vi "Actor Core.vi"(8 "error in":errorcluster, 11 "HardwareSetup_modle001:HardwareSetup_modle001":refnum<class "HardwareSetup_model001.lvclass">) -> (0 "error out":errorcluster, 3 "HardwareSetup_modle001:HardwareSetup_modle001":refnum<class "Actor.lvclass">)   [LabVIEW 2019, in "HardwareSetup_model001.lvlib" / "HardwareSetup_model001.lvclass"]
doc: "(<B>Filename</B>: Actor Framework.lvlib:Actor.lvclass:Actor Core.vi)\n\nReceives messages to the actor, reacts to them, and initiates any error handling that may shut the actor down.\n\nDescendant classes may override this VI to append parallel tasks for the actor to complete while it handles messages. Overrides use the Call Parent Method node."
uses:
  HardwareSetup_model001.lvclass
  PLC.ctl
  LIN.ctl
  CAN.ctl
  Programming.ctl
  DMM.ctl
  Scanner.ctl
  ElectronicLoad.ctl
  Oscilloscope.ctl
  Digital IO.ctl
  C:/Program Files (x86)/National Instruments/LabVIEW 2019/vi.lib/ActorFramework/Actor/Actor.lvclass
  <vilib>/ActorFramework/Actor/Actor.lvclass
  PowerSupply.ctl
  HardwareSetup_model001.lvclass/HardwareSetup_model001.ctl
  <vilib>/ActorFramework/Actor/Actor.lvclass/Actor.ctl
  <vilib>/ActorFramework/Message Enqueuer/Message Enqueuer.lvclass/Message Enqueuer.ctl
  2d133038-814c-4d09-b03d-156015606240.vi
  <vilib>/ActorFramework/Message Enqueuer/Init from Existing Queue.vi
  <vilib>/ActorFramework/Message Enqueuer/Enqueue.vi
  SystemSetup/SystemSetup Messages/RefreshSystemConfigurationUI Msg/RefreshSystemConfigurationUI Msg.lvclass
  C:/Program Files (x86)/National Instruments/LabVIEW 2019/vi.lib/ActorFramework/Message/Message.lvclass
  SystemSetup/SystemSetup Messages/SaveSystemConfigurationUI Msg/SaveSystemConfigurationUI Msg.lvclass
  <vilib>/ActorFramework/Message Priority Queue/Priority Enqueue.vi
  <vilib>/ActorFramework/Message Enqueuer/Message Enqueuer.lvclass
  SystemSetup/SystemSetup/SystemSetup.lvclass
  b9caf896-7e68-41be-8993-ec1cdb98c7cc.vi
  HardwareSetup_model001.lvlib
panel:
  in  "Tab Control":T1(tab)
  in  "PowerSupply":T2
  in  "Digital IO":T3
  in  "Oscilloscope":T4
  in  "ElectronicLoad":T5
  in  "Scanner":T6
  in  "DMM":T7
  in  "PLC":T8
  in  "CAN":T9
  in  "LIN":T10
  in  "Programming":T11
  in  "OK":bool
  in  "Cancel":bool
  # "PowerSupply_4"
  # "PowerSupply_3"
  # "PowerSupply_2"
  # "PowerSupply_1"
  # "Digital IO_4"
  # "Digital IO_3"
  # "Digital IO_2"
  # "Digital IO_1"
  # "Oscilloscope_4"
  # "Oscilloscope_3"
  # "Oscilloscope_2"
  # "Oscilloscope_1"
  # "ElectronicLoad_4"
  # "ElectronicLoad_3"
  # "ElectronicLoad_2"
  # "ElectronicLoad_1"
  # "Scanner_4"
  # "Scanner_3"
  # "Scanner_2"
  # "Scanner_1"
  # "DMM_4"
  # "DMM_3"
  # "DMM_2"
  # "DMM_1"
  # "PLC_1"
  # "CAN_4"
  # "CAN_3"
  # "CAN_2"
  # "CAN_1"
  # "LIN_4"
  # "LIN_3"
  # "LIN_2"
  # "LIN_1"
  # "Programming_1"
  # "Programming_1"
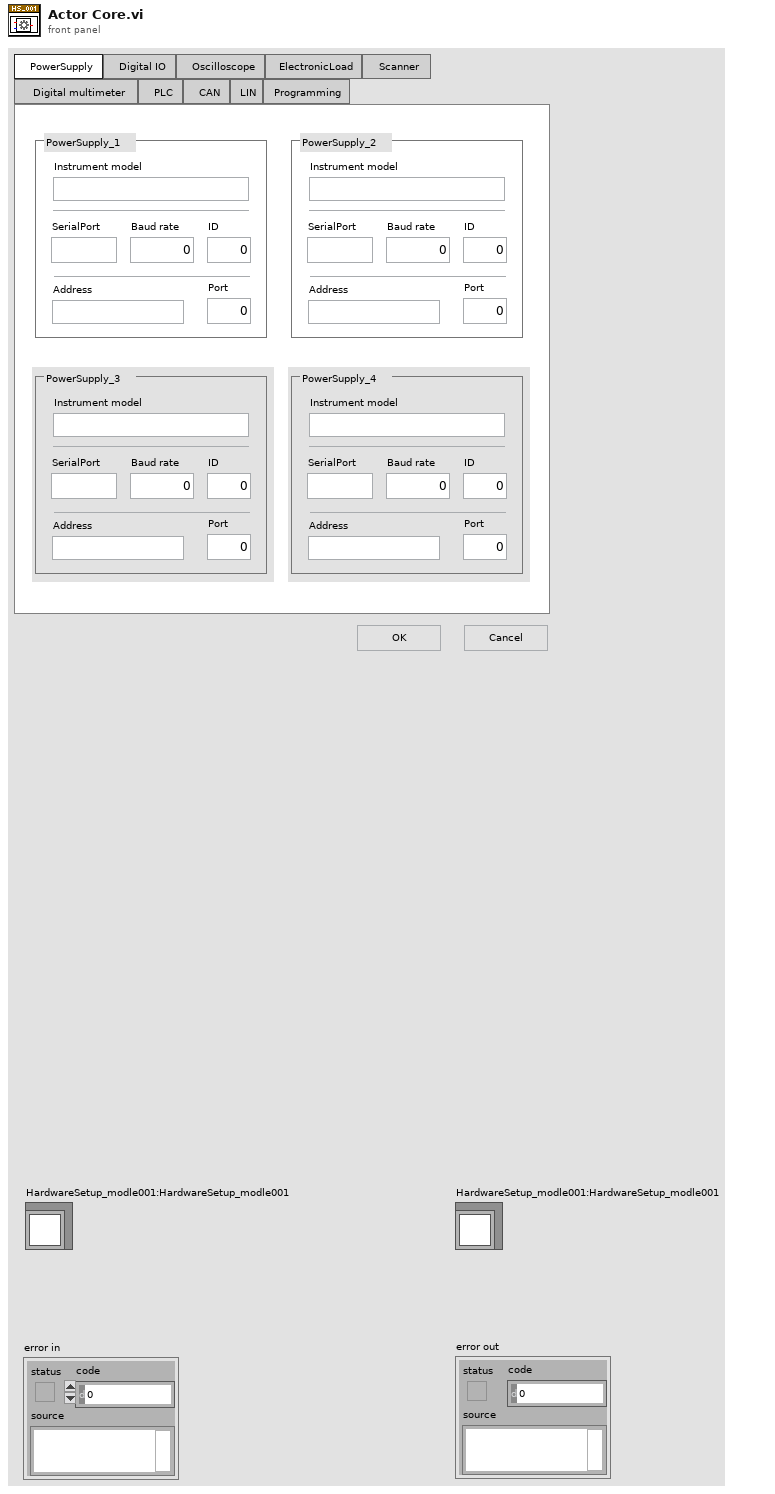
[diagram p1: front panel]
types:
  T1 = enum32{"  PowerSupply  ", "  Digital IO  ", "  Oscilloscope  ", "  ElectronicLoad ", "  Scanner   ", "  Digital multimeter    ", "  PLC  ", "  CAN  ", " LIN", " Programming "}
  T2 = typedef "HardwareSetup_model001.lvlib/PowerSupply.ctl" = cluster{"PowerSupply 1":cluster{"SerialPort":string, "Baud rate":i32, "Address":string, "ID":i32, "Port":i32, "Instrument model":string}, "PowerSupply 2":cluster{"SerialPort":string, "Baud rate":i32, "Address":string, "ID":i32, "Port":i32, "Instrument model":string}, "PowerSupply 3":cluster{"SerialPort":string, "Baud rate":i32, "Address":string, "ID":i32, "Port":i32, "Instrument model":string}, "PowerSupply 4":cluster{"SerialPort":string, "Baud rate":i32, "Address":string, "ID":i32, "Port":i32, "Instrument model":string}}
  T3 = typedef "HardwareSetup_model001.lvlib/Digital IO.ctl" = cluster{"Digital IO 1":cluster{"SerialPort":string, "Baud rate":i32, "Address":string, "ID":i32, "Port":i32, "Instrument model":string}, "Digital IO 2":cluster{"SerialPort":string, "Baud rate":i32, "Address":string, "ID":i32, "Port":i32, "Instrument model":string}, "Digital IO 3":cluster{"SerialPort":string, "Baud rate":i32, "Address":string, "ID":i32, "Port":i32, "Instrument model":string}, "Digital IO 4":cluster{"SerialPort":string, "Baud rate":i32, "Address":string, "ID":i32, "Port":i32, "Instrument model":string}}
  T4 = typedef "HardwareSetup_model001.lvlib/Oscilloscope.ctl" = cluster{"Oscilloscope 1":cluster{"SerialPort":string, "Baud rate":i32, "Address":string, "ID":i32, "Port":i32, "Instrument model":string}, "Oscilloscope 2":cluster{"SerialPort":string, "Baud rate":i32, "Address":string, "ID":i32, "Port":i32, "Instrument model":string}, "Oscilloscope 3":cluster{"SerialPort":string, "Baud rate":i32, "Address":string, "ID":i32, "Port":i32, "Instrument model":string}, "Oscilloscope 4":cluster{"SerialPort":string, "Baud rate":i32, "Address":string, "ID":i32, "Port":i32, "Instrument model":string}}
  T5 = typedef "HardwareSetup_model001.lvlib/ElectronicLoad.ctl" = cluster{"ElectronicLoad 1":cluster{"SerialPort":string, "Baud rate":i32, "Address":string, "ID":i32, "Port":i32, "Instrument model":string}, "ElectronicLoad 2":cluster{"SerialPort":string, "Baud rate":i32, "Address":string, "ID":i32, "Port":i32, "Instrument model":string}, "ElectronicLoad 3":cluster{"SerialPort":string, "Baud rate":i32, "Address":string, "ID":i32, "Port":i32, "Instrument model":string}, "ElectronicLoad 4":cluster{"SerialPort":string, "Baud rate":i32, "Address":string, "ID":i32, "Port":i32, "Instrument model":string}}
  T6 = typedef "HardwareSetup_model001.lvlib/Scanner.ctl" = cluster{"Scanner 1":cluster{"SerialPort":string, "Baud rate":i32, "Address":string, "ID":i32, "Port":i32, "Instrument model":string}, "Scanner 2":cluster{"SerialPort":string, "Baud rate":i32, "Address":string, "ID":i32, "Port":i32, "Instrument model":string}, "Scanner 3":cluster{"SerialPort":string, "Baud rate":i32, "Address":string, "ID":i32, "Port":i32, "Instrument model":string}, "Scanner 4":cluster{"SerialPort":string, "Baud rate":i32, "Address":string, "ID":i32, "Port":i32, "Instrument model":string}}
  T7 = typedef "HardwareSetup_model001.lvlib/DMM.ctl" = cluster{"DMM 1":cluster{"SerialPort":string, "Baud rate":i32, "Address":string, "ID":i32, "Port":i32, "Instrument model":string}, "DMM 2":cluster{"SerialPort":string, "Baud rate":i32, "Address":string, "ID":i32, "Port":i32, "Instrument model":string}, "DMM 3":cluster{"SerialPort":string, "Baud rate":i32, "Address":string, "ID":i32, "Port":i32, "Instrument model":string}, "DMM 4":cluster{"SerialPort":string, "Baud rate":i32, "Address":string, "ID":i32, "Port":i32, "Instrument model":string}}
  T8 = typedef "HardwareSetup_model001.lvlib/PLC.ctl" = cluster{"PLC 1":cluster{"SerialPort":string, "Baud rate":i32, "Address":string, "ID":i32, "Port":i32, "Instrument model":string}}
  T9 = typedef "HardwareSetup_model001.lvlib/CAN.ctl" = cluster{"CAN 1":cluster{"Instrument model":string, "Port":string, "Baud rate":i32, "ID":i32, "Terminal":bool}, "CAN 2":cluster{"Instrument model":string, "Port":string, "Baud rate":i32, "ID":i32, "Terminal":bool}, "CAN 3":cluster{"Instrument model":string, "Port":string, "Baud rate":i32, "ID":i32, "Terminal":bool}, "CAN 4":cluster{"Instrument model":string, "Port":string, "Baud rate":i32, "ID":i32, "Terminal":bool}}
  T10 = typedef "HardwareSetup_model001.lvlib/LIN.ctl" = cluster{"LIN 1":cluster{"Instrument model":string, "Port":string, "Baud rate":i32, "ID":i32, "Terminal":bool}, "LIN 2":cluster{"Instrument model":string, "Port":string, "Baud rate":i32, "ID":i32, "Terminal":bool}, "LIN 3":cluster{"Instrument model":string, "Port":string, "Baud rate":i32, "ID":i32, "Terminal":bool}, "LIN 4":cluster{"Instrument model":string, "Port":string, "Baud rate":i32, "ID":i32, "Terminal":bool}}
  T11 = typedef "HardwareSetup_model001.lvlib/Programming.ctl" = cluster{"Programming 1":cluster{"Test Image":string, "Address":string, "Port":i32, "Instrument model":string, "Final Image":string}, "Programming 2":cluster{"Test Image":string, "Address":string, "Port":i32, "Instrument model":string, "Final Image":string}}
  T12 = enum32{"Invalid", "Standard", "Closed", "Hidden", "Minimized", "Maximized"}
  T13 = enum32{"invalid app kind", "Development System", "Run Time System", "Student Edition", "Embedded LabVIEW", "Evaluation", "Custom"}
  T14 = cluster{"Core":cluster{"Current VI Reference":refnum<vi>, "Close Panel on Exit?":bool}, "Your Boolean data":bool, "Your string data":string}
  T15 = cluster{"Current VI Reference":refnum<vi>, "Close Panel on Exit?":bool}
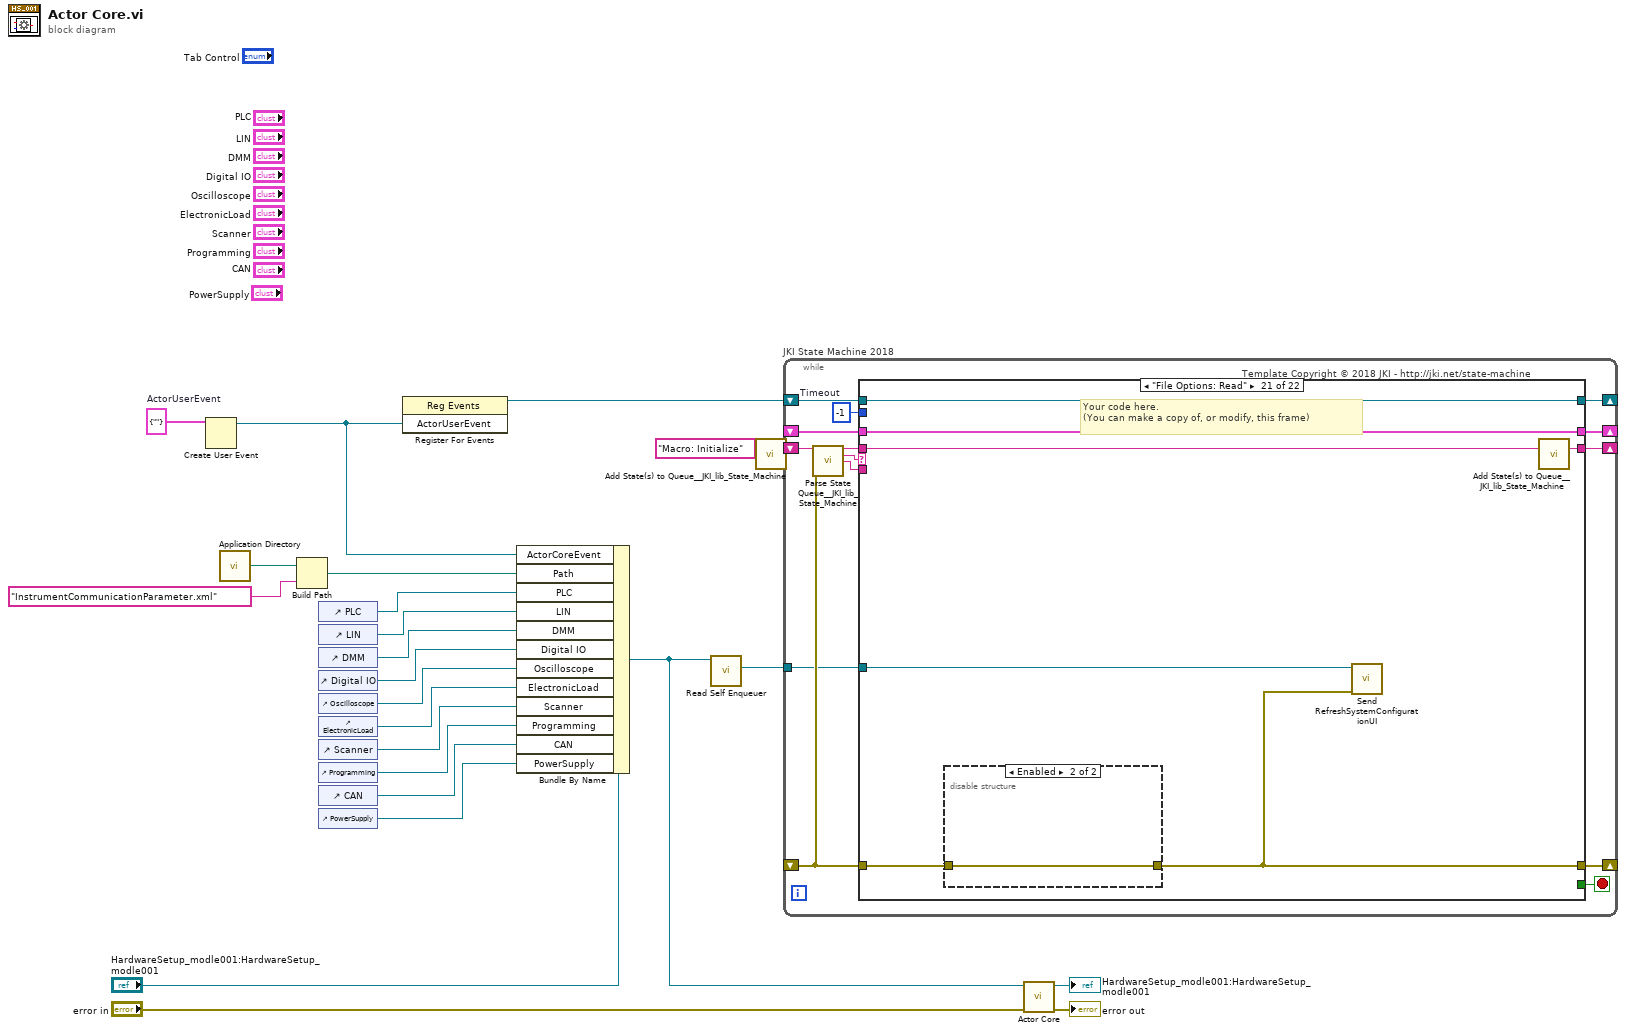
[diagram p0: block diagram]
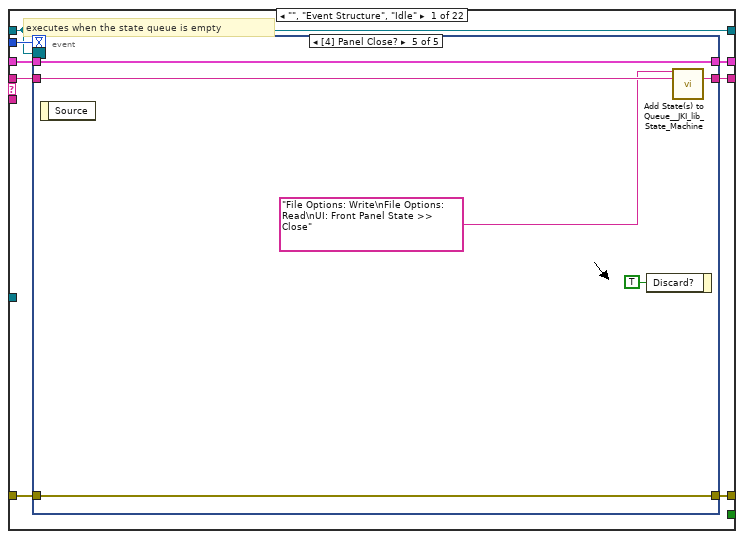
[diagram p2: hidden frame]
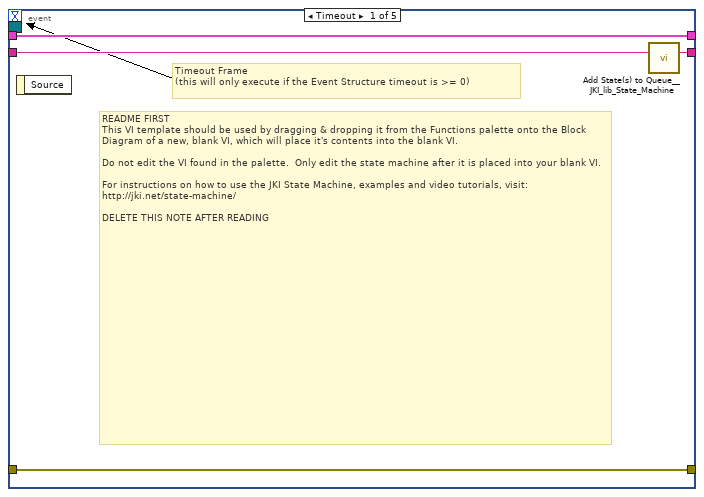
[diagram p3: hidden frame]
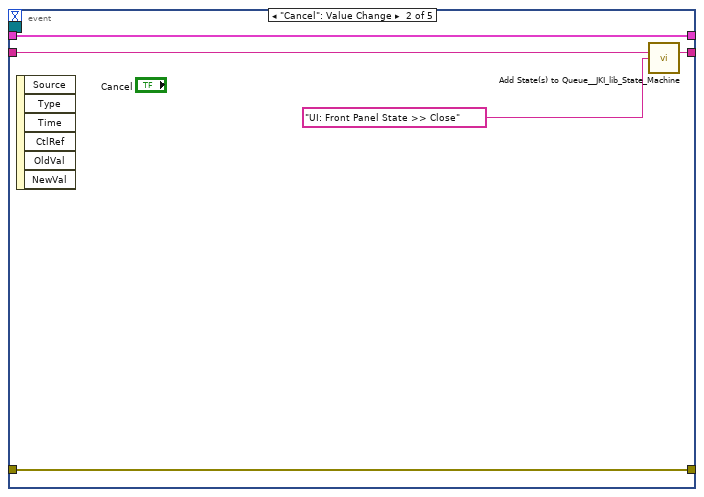
[diagram p4: hidden frame]
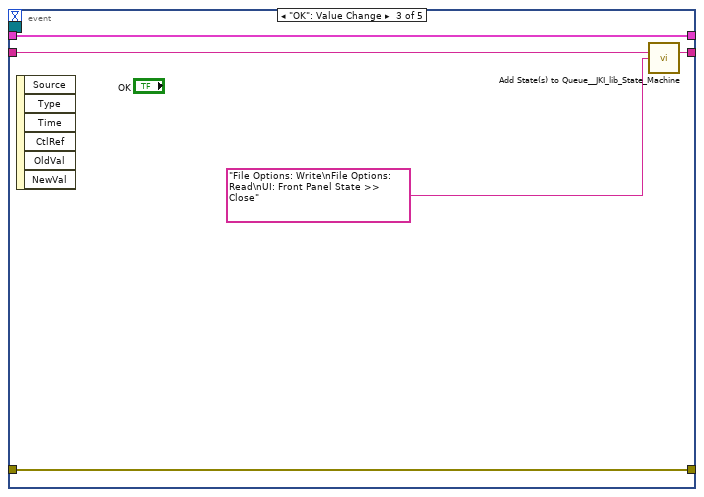
[diagram p5: hidden frame]
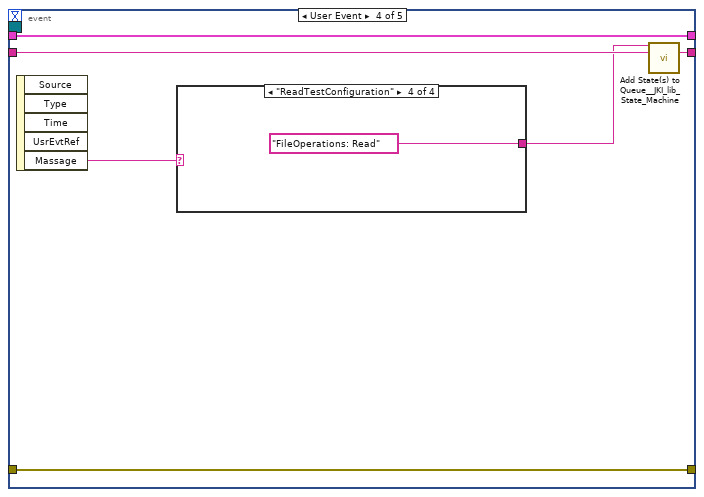
[diagram p6: hidden frame]
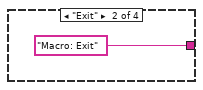
[diagram p8: hidden frame]
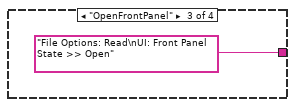
[diagram p9: hidden frame]
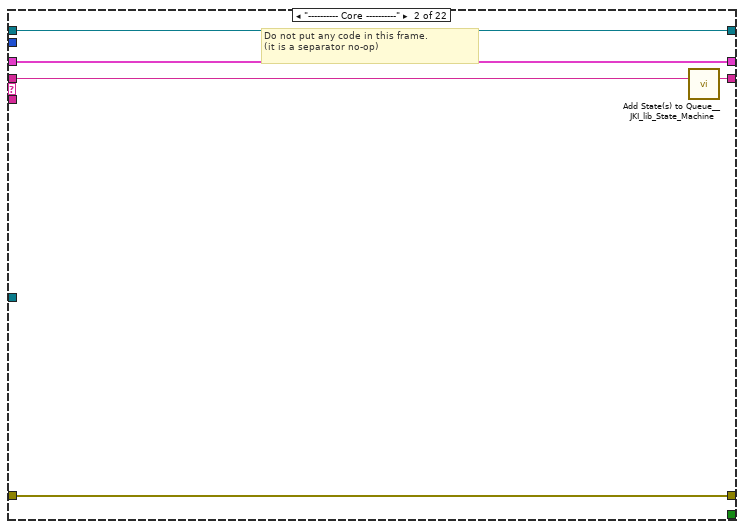
[diagram p10: hidden frame]
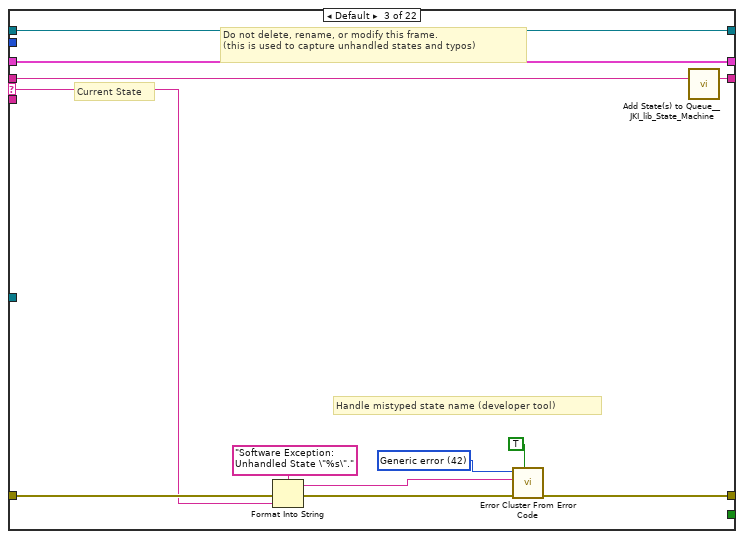
[diagram p11: hidden frame]
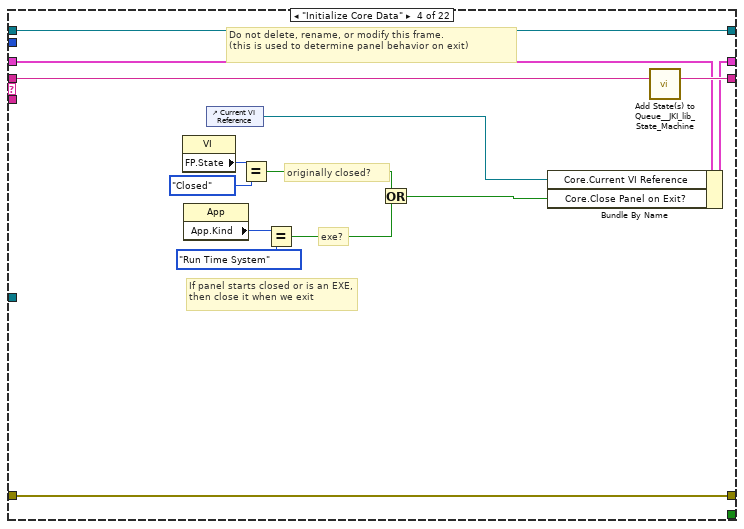
[diagram p12: hidden frame]
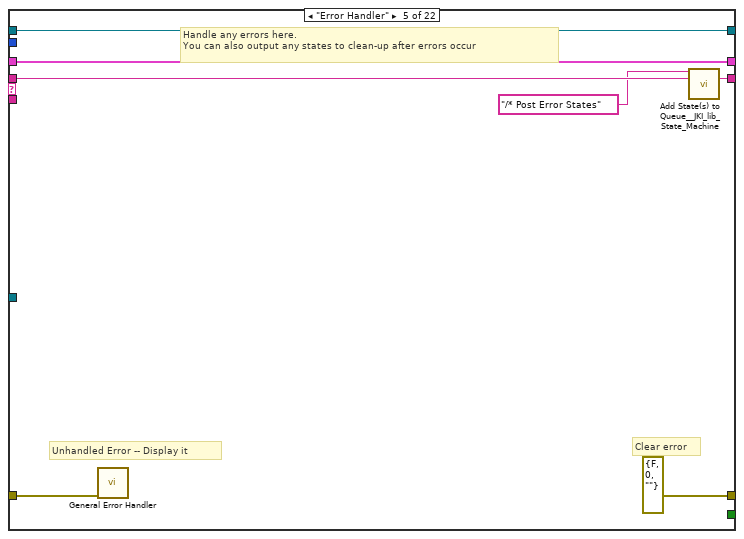
[diagram p13: hidden frame]
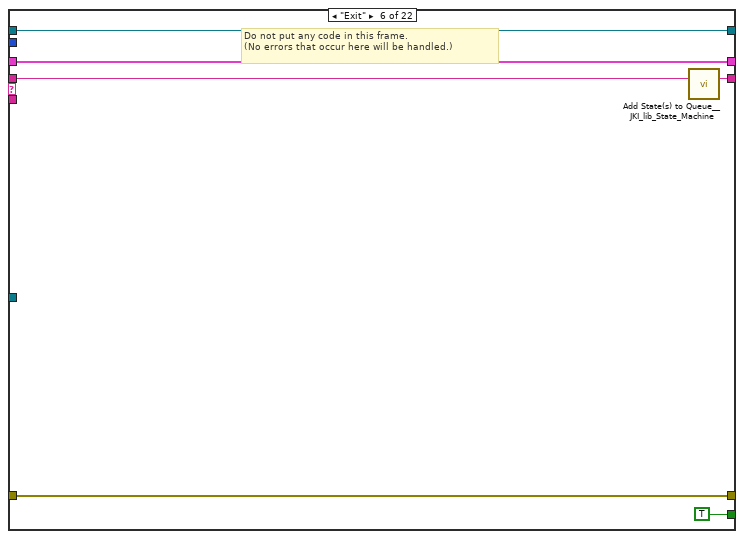
[diagram p14: hidden frame]
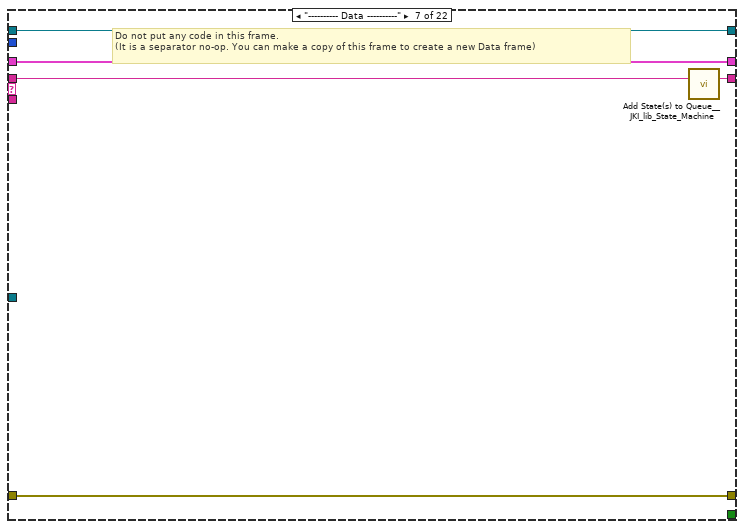
[diagram p15: hidden frame]
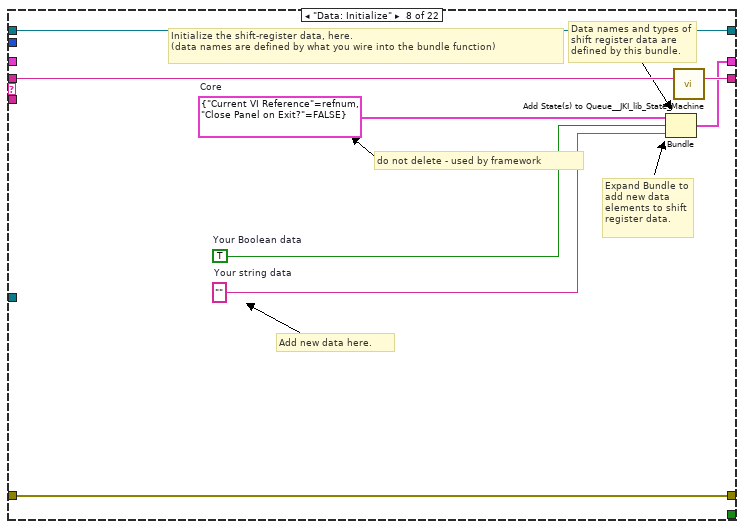
[diagram p16: hidden frame]
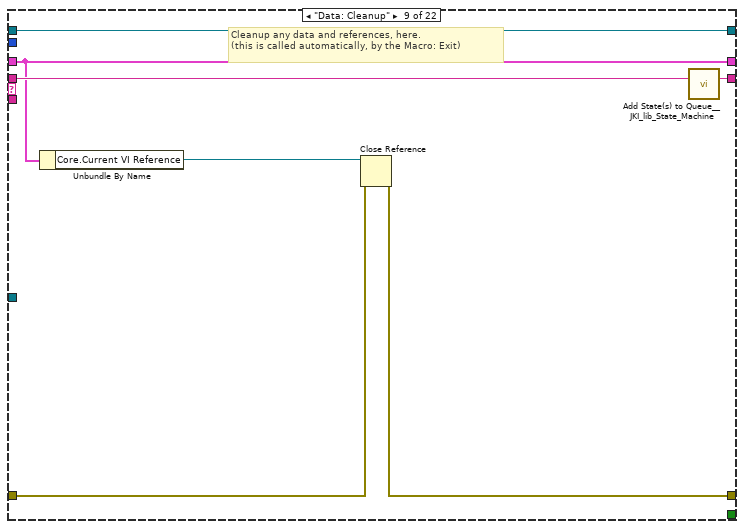
[diagram p17: hidden frame]
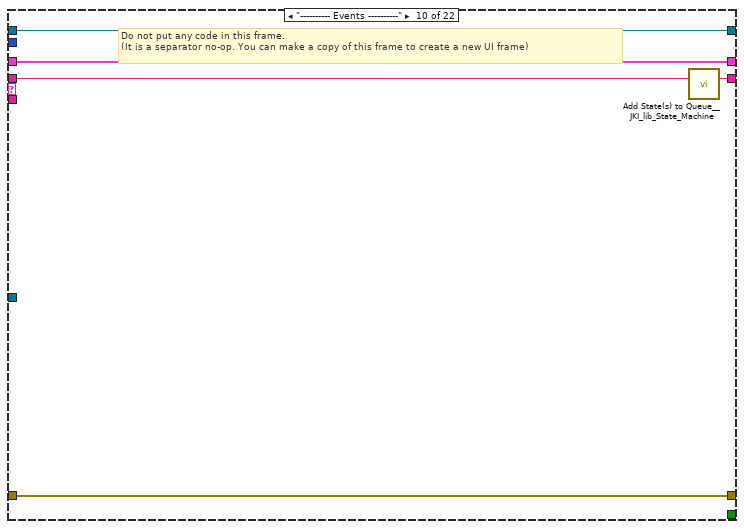
[diagram p18: hidden frame]
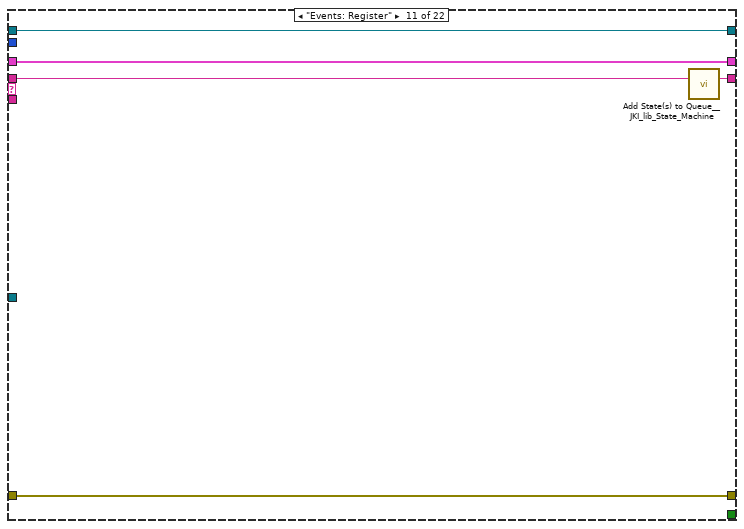
[diagram p19: hidden frame]
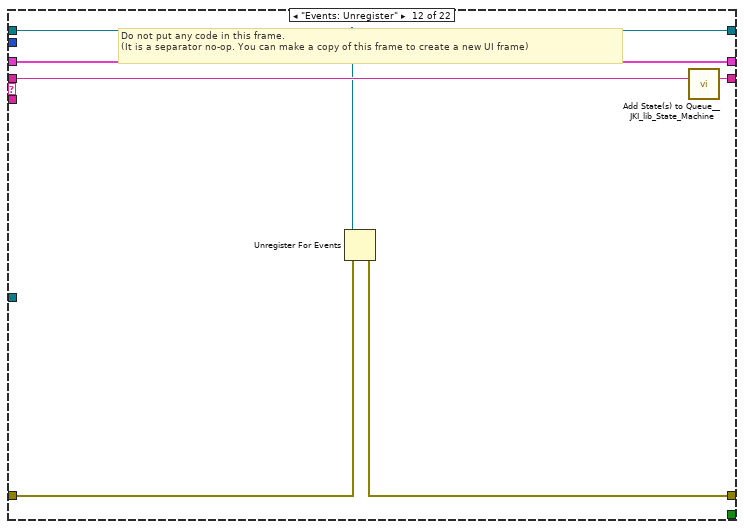
[diagram p20: hidden frame]
diagram:
  w19 = cluster{"Massage":string} {"Massage"=""}  # ActorUserEvent
  n1 = Create User Event(user event datatype=w19) -> (user event=w17:refnum<user-event>)  [unwired: 1 in, 1 out]
  n2 = call <vilib>:"Application Directory.vi"() -> ("Application Directory"=w15:path)
  n3 = Build Path(base path=w15, name or relative path="InstrumentCommunicationParameter.xml") -> (appended path=w11:path)
  n4 = control-ref of="PLC"() -> (w10:refnum<vi>)
  n5 = control-ref of="LIN"() -> (w9:refnum<vi>)
  n6 = control-ref of="DMM"() -> (w8:refnum<vi>)
  n7 = control-ref of="Digital IO"() -> (w7:refnum<vi>)
  n8 = control-ref of="Oscilloscope"() -> (w6:refnum<vi>)
  n9 = control-ref of="ElectronicLoad"() -> (w5:refnum<vi>)
  n10 = control-ref of="Scanner"() -> (w4:refnum<vi>)
  n11 = control-ref of="Programming"() -> (w3:refnum<vi>)
  n12 = control-ref of="CAN"() -> (w2:refnum<vi>)
  n13 = control-ref of="PowerSupply"() -> (w1:refnum<vi>)
  n14 = register-events(w17) -> (reference out=w18:refnum<event-registration>)  [unwired: 2 in, 1 out]
  n15 = Bundle By Name(cluster="HardwareSetup_modle001:HardwareSetup_modle001", "ActorCoreEvent"=w17, "Path"=w11, "PLC"=w10, "LIN"=w9, "DMM"=w8, "Digital IO"=w7, "Oscilloscope"=w6, "ElectronicLoad"=w5, "Scanner"=w4, "Programming"=w3, "CAN"=w2, "PowerSupply"=w1) -> (w12:refnum<class "HardwareSetup_model001.lvclass">)
  n16 = call <vilib>:"Read Self Enqueuer.vi"("Actor"=w12) -> ("Self Enqueuer"=w16:refnum<class "Message Enqueuer.lvclass">)  [unwired: 10 in]
  n17 = call <vilib>:"Add State(s) to Queue__JKI_lib_State_Machine.vi"("State(s) in (\"\")"="Macro: Initialize") -> ("States Out"=w21:string)  [unwired: 14 in]
  n18 = while "JKI State Machine 2018" {
    shift-right: [w31] -> _
    shift-left: _ -> [w30]
    shift-right: [w34] -> _
    shift-left: _ -> [w28]
    shift-right: [w33] -> _
    shift-left: w21 -> [w35]
    shift-right: [w27] -> _
    shift-left: w18 -> [w26]
    tunnel: w16 -> [w25]
    stop <- w32 stop-if-true
    w29 = -1  # Timeout
    # "Template Copyright © 2018 JKI - http://jki.net/state-machine"
    n19 = call <vilib>:"Parse State Queue__JKI_lib_State_Machine.vi"("State Queue"=w35, "Error In (no error)"=w28) -> ("Remaining States"=w37:string, "Current State"=w38:string, "Arguments"=w36:string)  [unwired: 11 in]
    n20 = case shown="\"File Options: Read\"" w38 {
      selector: w38 -> [_ _ w82 _ _ _ _ _ _ _ _ _ _ _ _ _ _ _ _ _ _ _]
      tunnel: w37 -> [w46 w80 w86 w106 w113 w119 w124 w132 w139 w144 w149 w155 w160 w167 w174 w186 w256 w262 w273 w278 w285 w298]
      tunnel: w36 -> [_ _ _ _ _ _ _ _ _ _ _ _ _ _ w169 w180 _ _ _ _ _ _]
      tunnel: w30 -> [w44 w77 w84 w99 w110 w117 w121 _ w134 w141 w147 w153 w157 w165 w172 w182 w253 w259 w270 w275 w283 w295]
      tunnel: [w43 w78 w88 w103 errorcluster {"status"=FALSE, "code"=0, "source"=""} ("error out") w116 w122 w129 w135 w142 w145 w150 w158 w161 w170 w183 w254 w260 w271 w276 w279 w296] -> w34
      tunnel: w28 -> [w42 w78 w87 w103 w109 w116 w122 w129 w136 w142 w145 w151 w158 w162 w171 w184 w254 w260 w271 w276 w280 w296]
      tunnel: [w45 w79 w85 w105 w112 w118 w123 w131 w138 w143 w148 w154 w159 w166 w173 w185 w255 w261 w272 w277 w284 w297] -> w33
      tunnel: [_ _ _ _ _ TRUE _ _ _ _ _ _ _ _ _ _ _ _ _ _ _ _] -> w32
      tunnel: [w41 w77 w84 w104 w110 w117 w121 w130 w134 w141 w147 w153 w157 w165 w172 w182 w253 w259 w270 w275 w283 w295] -> w31
      tunnel: w29 -> [w40 _ _ _ _ _ _ _ _ _ _ _ _ _ _ _ _ _ _ _ _ _]
      tunnel: [w39 w76 w81 w93 w107 w114 w120 w125 w133 w140 w146 w152 w156 w164 w168 w179 w252 w257 w263 w274 w282 w294] -> w27
      tunnel: w26 -> [w39 w76 w81 w93 w107 w114 w120 w125 w133 w140 w146 w152 w156 w164 w168 w179 w252 w257 w263 w274 w282 w294]
      tunnel: w25 -> [_ _ _ _ _ _ _ _ _ _ _ _ _ _ _ _ _ _ _ _ w281 w293]
      frame "", "Event Structure", "Idle" {
        # "executes when the state queue is empty"
        n21 = event shown="[4] Panel Close?" {
          selector: w39 -> [_ _ _ _ _]
          dyn-events: _ -> [_ _ _ _ _]
          timeout: w40 -> [_ _ _ _ _]
          tunnel: w46 -> [w50 w55 w60 w66 w75]
          tunnel: [w49 w54 w59 w65 w74] -> w45
          tunnel: w44 -> [w47 w52 w57 w63 w72]
          tunnel: [w48 w53 w58 w64 w73] -> w43
          tunnel: w42 -> [w48 w53 w58 w64 w73]
          tunnel: [w47 w52 w57 w63 w72] -> w41
          event Timeout {
            # "README FIRST\nThis VI template should be used by dragging & dropping it from the Functions palette onto the Block Diagram of a new, blank VI, which will place it's contents into the blank VI.\n\nDo not edit the VI found in the palette.  Only edit the state machine after it is placed into your blank VI.\n\nFor instructions on how to use the JKI State Machine, examples and video tutorials, visit:\nhttp://jki.net/state-machine/\n\nDELETE THIS NOTE AFTER READING"
            # "Timeout Frame\n(this will only execute if the Event Structure timeout is >= 0)"
            n22 = event-data() -> ()  [unwired: 1 in, 1 out]
            n23 = call <vilib>:"Add State(s) to Queue__JKI_lib_State_Machine.vi"("State(s) in (\"\")"=w50) -> ("States Out"=w49:string)  [unwired: 14 in]
          }
          event "Cancel": Value Change {
            n24 = event-data() -> ()  [unwired: 1 in, 6 out]
            n25 = call <vilib>:"Add State(s) to Queue__JKI_lib_State_Machine.vi"("State(s) in (\"\")"=w55, "State(s) at Back (\"\")"="UI: Front Panel State >> Close") -> ("States Out"=w54:string)  [unwired: 13 in]
          }
          event "OK": Value Change {
            n26 = event-data() -> ()  [unwired: 1 in, 6 out]
            n27 = call <vilib>:"Add State(s) to Queue__JKI_lib_State_Machine.vi"("State(s) in (\"\")"=w60, "State(s) at Back (\"\")"="File Options: Write\nFile Options: Read\nUI: Front Panel State >> Close") -> ("States Out"=w59:string)  [unwired: 13 in]
          }
          event User Event {
            n28 = event-data() -> ("Massage"=w62:string)  [unwired: 1 in, 4 out]
            n29 = case shown="\"ReadTestConfiguration\"" w62 {
              tunnel: [_ "Macro: Exit" "File Options: Read\nUI: Front Panel State >> Open" "FileOperations: Read"] -> w61
              frame "Idle", Default {
              }
              frame "Exit" {
              }
              frame "OpenFrontPanel" {
              }
              frame "ReadTestConfiguration" {
              }
            }
            n30 = call <vilib>:"Add State(s) to Queue__JKI_lib_State_Machine.vi"("State(s) in Front (\"\")"=w61, "State(s) in (\"\")"=w66) -> ("States Out"=w65:string)  [unwired: 13 in]
          }
          event Panel Close? {
            n31 = event-data() -> ()  [unwired: 1 in, 1 out]
            n32 = event-data("Discard?"=TRUE) -> ()  [unwired: 1 in, 1 out]
            n33 = call <vilib>:"Add State(s) to Queue__JKI_lib_State_Machine.vi"("State(s) in Front (\"\")"="File Options: Write\nFile Options: Read\nUI: Front Panel State >> Close", "State(s) in (\"\")"=w75) -> ("States Out"=w74:string)  [unwired: 13 in]
          }
        }
      }
      frame "---------- Core ----------" {
        # "Do not put any code in this frame.\n(it is a separator no-op)"
        n34 = call <vilib>:"Add State(s) to Queue__JKI_lib_State_Machine.vi"("State(s) in (\"\")"=w80) -> ("States Out"=w79:string)  [unwired: 14 in]
      }
      frame Default {
        w91 = 42 items=["No error", "Argument error", "Memory is full", "Out of zone", "End of file", "File already open", "Generic file I/O error", "File not found", "File permission error", "Disk is full", "Duplicate path", "Too many files open", "System feature not enabled", "Resource file not found", "Cannot add resource", "Resource not found", "Image not found", "Image memory error", "Pen does not exist", "Config type invalid", "Config token not found", "Config parse error", "Config memory error", "Bad external code format", "Bad external code offset", "External code not present", "Null window", "Destroy window error", "Null menu", "Print aborted", "Bad print record", "Print driver error", "Windows error during printing", "Memory error during printing", "Print dialog error", "Generic print error", "Invalid device refnum", "Device not found", "Device parameter error", "Device unit error", "Cannot open device", "Device call aborted", "Generic error", "Cancelled by user", "Object ID too low", "Object ID too high", "Object not in heap", "Unknown heap", "Unknown object (invalid DefProc)", "Unknown object (DefProc not in table)", "Message out of range", "Invalid (null) method", "Unknown message", "Manager call not supported", "Bad address", "Network operation in progress", "Network operation timed out", "Connection is busy", "Network attribute not supported", "Network error", "Address in use", "System out of memory", "Connection aborted", "Connection refused", "Not connected", "Already connected", "Connection closed", "Initialization error (interapplication manager)", "Bad occurrence", "Wait on unbound occurrence handler", "Occurrence queue overflow", "Datalog type conflict", "Unused", "Unrecognized type (interapplication manager)", "Memory corrupt", "Failed to make temporary DLL", "Old CIN version", "Drag socket not found", "Failed to load drop-object", "Failed to register OLE object", "Failed to release OLE object", "Format specifier type mismatch", "Unknown format specifier", "Too few format specifiers", "Too many format specifiers", "Scan failed", "Newer CIN version", "Error converting to variant", "Runtime menu error", "Password tampered", "Variant attribute not found", "Incompatible variant data type", "Event data is not available", "Event Store is not present", "Occurrence is not found", "Event Queue is not created", "Event info is not available", "Refnum passed is NULL", "Error retrieving Class GUID", "Error retrieving CoClass GUID", "Error retrieving TypeLib GUID.", "Bad built application magic bytes.", "Specific driver is different from the specific driver associated with the Logical Name.", "There is no session opened to the class driver.", "Max Error", "MAX - Error with config objects", "MAX - Error loading configuration", "MAX - Group not supported"]
        # "Current State"
        # "Do not delete, rename, or modify this frame.\n(this is used to capture unhandled states and typos)"
        # "Handle mistyped state name (developer tool)"
        n35 = Format Into String(format string="Software Exception: Unhandled State \"%s\"." ("message"), error in=w87, w82) -> (resulting string=w90:string, error out=w89:errorcluster)  [unwired: 1 in]
        n36 = call <vilib>:"Error Cluster From Error Code.vi"("show call chain? (False)"=TRUE, "error in (no error)"=w89, "error message (\"\")"=w90, "error code (0)"=w91) -> ("error out"=w88:errorcluster)  [unwired: 5 in]
        n37 = call <vilib>:"Add State(s) to Queue__JKI_lib_State_Machine.vi"("State(s) in (\"\")"=w86) -> ("States Out"=w85:string)  [unwired: 14 in]
      }
      frame "Initialize Core Data" {
        # "Do not delete, rename, or modify this frame.\n(this is used to determine panel behavior on exit)"
        # "originally closed?"
        # "exe?"
        # "If panel starts closed or is an EXE, then close it when we exit"
        n38 = property class="VI"() -> ("FP.State"=w96:T12)  [unwired: 2 in, 2 out]
        n39 = property class="App"() -> ("App.Kind"=w102:T13)  [unwired: 2 in, 2 out]
        n40 = control-ref of="Current VI Reference"() -> (w97:refnum<vi>)
        n41 = Equal?(x=w96, y=T12."Closed" ("Front Panel Window:State")) -> (x = y?=w94:bool)
        n42 = Equal?(x=w102, y=T13."Run Time System" ("Application:Kind")) -> (x = y?=w100:bool)
        n43 = Or(x=w94, y=w100) -> (x .or. y?=w98:bool)
        n44 = Bundle By Name(cluster=w99, "Core.Current VI Reference"=w97, "Core.Close Panel on Exit?"=w98) -> (w104:T14)
        n45 = call <vilib>:"Add State(s) to Queue__JKI_lib_State_Machine.vi"("State(s) in (\"\")"=w106) -> ("States Out"=w105:string)  [unwired: 14 in]
      }
      frame "Error Handler" {
        # "Unhandled Error -- Display it"
        # "Handle any errors here.\nYou can also output any states to clean-up after errors occur"
        # "Clear error"
        n46 = call <vilib>:"General Error Handler.vi"("error in (no error)"=w109) -> ()  [unwired: 10 in, 5 out]
        n47 = call <vilib>:"Add State(s) to Queue__JKI_lib_State_Machine.vi"("State(s) in Front (\"\")"="/* Post Error States", "State(s) in (\"\")"=w113) -> ("States Out"=w112:string)  [unwired: 13 in]
      }
      frame "Exit" {
        # "Do not put any code in this frame.\n(No errors that occur here will be handled.)"
        n48 = call <vilib>:"Add State(s) to Queue__JKI_lib_State_Machine.vi"("State(s) in (\"\")"=w119) -> ("States Out"=w118:string)  [unwired: 14 in]
      }
      frame "---------- Data ----------" {
        # "Do not put any code in this frame.\n(It is a separator no-op. You can make a copy of this frame to create a new Data frame)"
        n49 = call <vilib>:"Add State(s) to Queue__JKI_lib_State_Machine.vi"("State(s) in (\"\")"=w124) -> ("States Out"=w123:string)  [unwired: 14 in]
      }
      frame "Data: Initialize" {
        w126 = T15 {"Current VI Reference"=refnum, "Close Panel on Exit?"=FALSE}  # Core
        w128 = TRUE  # Your Boolean data
        w127 = ""  # Your string data
        # "do not delete - used by framework"
        # "Expand Bundle to add new data elements to shift register data."
        # "Add new data here."
        # "Data names and types of shift register data are defined by this bundle."
        # "Initialize the shift-register data, here.\n(data names are defined by what you wire into the bundle function)"
        n50 = Bundle("Core"=w126, "Your Boolean data"=w128, "Your string data"=w127) -> (w130:T14)  [unwired: 1 in]
        n51 = call <vilib>:"Add State(s) to Queue__JKI_lib_State_Machine.vi"("State(s) in (\"\")"=w132) -> ("States Out"=w131:string)  [unwired: 14 in]
      }
      frame "Data: Cleanup" {
        # "Cleanup any data and references, here.\n(this is called automatically, by the Macro: Exit)"
        n52 = Unbundle By Name(w134) -> ("Core.Current VI Reference"=w137:refnum<vi>)
        n53 = Close Reference(reference=w137, error in (no error)=w136) -> (error out=w135:errorcluster)
        n54 = call <vilib>:"Add State(s) to Queue__JKI_lib_State_Machine.vi"("State(s) in (\"\")"=w139) -> ("States Out"=w138:string)  [unwired: 14 in]
      }
      frame "---------- Events ----------" {
        # "Do not put any code in this frame.\n(It is a separator no-op. You can make a copy of this frame to create a new UI frame)"
        n55 = call <vilib>:"Add State(s) to Queue__JKI_lib_State_Machine.vi"("State(s) in (\"\")"=w144) -> ("States Out"=w143:string)  [unwired: 14 in]
      }
      frame "Events: Register" {
        n56 = call <vilib>:"Add State(s) to Queue__JKI_lib_State_Machine.vi"("State(s) in (\"\")"=w149) -> ("States Out"=w148:string)  [unwired: 14 in]
      }
      frame "Events: Unregister" {
        # "Do not put any code in this frame.\n(It is a separator no-op. You can make a copy of this frame to create a new UI frame)"
        n57 = Unregister For Events(event registration refnum=w152, error in=w151) -> (error out=w150:errorcluster)
        n58 = call <vilib>:"Add State(s) to Queue__JKI_lib_State_Machine.vi"("State(s) in (\"\")"=w155) -> ("States Out"=w154:string)  [unwired: 14 in]
      }
      frame "---------- UI ----------" {
        # "Do not put any code in this frame.\n(It is a separator no-op. You can make a copy of this frame to create a new UI frame)"
        n59 = call <vilib>:"Add State(s) to Queue__JKI_lib_State_Machine.vi"("State(s) in (\"\")"=w160) -> ("States Out"=w159:string)  [unwired: 14 in]
      }
      frame "UI: Initialize" {
        # "Initialize the User Interface, here.\n(this is called automatically, by the Macro: Init)"
        n60 = call "Stall Data Flow.vim"("value in"=w162, "milliseconds to wait"=u32 900) -> ("value out"=w161:errorcluster)  [unwired: 1 out]
        n61 = call <vilib>:"Add State(s) to Queue__JKI_lib_State_Machine.vi"("State(s) in (\"\")"=w167) -> ("States Out"=w166:string)  [unwired: 14 in]
      }
      frame "UI: Cursor Set" {
        # "Argument"
        # "Set and Unset Cursor Busy.\n(Usage: \"UI: Cursor Set >> Busy|Idle\")"
        n62 = case shown="\"Idle\", Default" w169 {
          tunnel: w171 -> [w176 w178]
          tunnel: [w175 w177] -> w170
          frame "Idle", Default {
            n63 = call <vilib>:"Unset Busy.vi"("error in (no error)"=w176) -> ("error out"=w175:errorcluster)  [unwired: 10 in]
          }
          frame "Busy" {
            n64 = call <vilib>:"Set Busy.vi"("error in (no error)"=w178) -> ("error out"=w177:errorcluster)  [unwired: 9 in, 1 out]
          }
        }
        n65 = call <vilib>:"Add State(s) to Queue__JKI_lib_State_Machine.vi"("State(s) in (\"\")"=w174) -> ("States Out"=w173:string)  [unwired: 14 in]
      }
      frame "UI: Front Panel State" {
        # "Argument"
        # "Set Front Panel Open or Closed\n(Usage: \"UI: Front Panel State >> Open|Close\")"
        n66 = Unbundle By Name(w182) -> ("Core.Current VI Reference"=w181:refnum<vi>)
        n67 = case shown="\"Maximize\", \"Maximized\"" w180 {
          tunnel: w184 -> [w192 w207 w218 w231 w244]
          tunnel: [w194 w208 w220 w233 w246] -> w183
          tunnel: w181 -> [w193 w205 w219 w232 w245]
          frame "Open", "Standard", Default {
            w187 = T12."Standard" ("State")
            n68 = property class="VI"(reference=w193, error in=w192) -> (reference out=w190:refnum<vi>, error out=w191:errorcluster, "FP.State"=w189:T12)
            n69 = Not Equal?(x=w189, y=w187) -> (x != y?=w188:bool)
            n70 = case shown="True" w188 {
              tunnel: [w198 w200] -> w194
              tunnel: w191 -> [w197 w200]
              tunnel: w190 -> [w196 _]
              tunnel: w187 -> [w195 _]
              frame True {
                n71 = invoke class="VI" method="FP.Open"(reference=w196, error in=w197, "Activate"=TRUE, "State"=w195) -> (error out=w198:errorcluster)  [unwired: 1 in, 4 out]
              }
              frame False {
              }
            }
          }
          frame "Close", "Closed" {
            n72 = property class="VI"(reference=w205, error in=w207) -> (reference out=w204:refnum<vi>, error out=w206:errorcluster, "FP.State"=w202:T12)
            n73 = Not Equal?(x=w202, y=T12."Closed" ("Front Panel Window:State")) -> (x != y?=w201:bool)
            n74 = case shown="True" w201 {
              tunnel: [w209 w212] -> w208
              tunnel: w206 -> [w209 w211]
              tunnel: w204 -> [_ w210]
              frame False {
              }
              frame True {
                n75 = invoke class="VI" method="FP.Close"(reference=w210, error in=w211) -> (error out=w212:errorcluster)  [unwired: 1 in, 2 out]
              }
            }
          }
          frame "Hidden", "Hide" {
            w213 = T12."Hidden" ("State")
            n76 = property class="VI"(reference=w219, error in=w218) -> (reference out=w216:refnum<vi>, error out=w217:errorcluster, "FP.State"=w215:T12)
            n77 = Not Equal?(x=w215, y=w213) -> (x != y?=w214:bool)
            n78 = case shown="True" w214 {
              tunnel: [w224 w225] -> w220
              tunnel: w217 -> [w223 w225]
              tunnel: w216 -> [w222 _]
              tunnel: w213 -> [w221 _]
              frame True {
                n79 = invoke class="VI" method="FP.Open"(reference=w222, error in=w223, "State"=w221) -> (error out=w224:errorcluster)  [unwired: 2 in, 4 out]
              }
              frame False {
              }
            }
          }
          frame "Minimize", "Minimized" {
            w226 = T12."Minimized" ("State")
            n80 = property class="VI"(reference=w232, error in=w231) -> (reference out=w229:refnum<vi>, error out=w230:errorcluster, "FP.State"=w228:T12)
            n81 = Not Equal?(x=w228, y=w226) -> (x != y?=w227:bool)
            n82 = case shown="True" w227 {
              tunnel: [w237 w238] -> w233
              tunnel: w230 -> [w236 w238]
              tunnel: w229 -> [w235 _]
              tunnel: w226 -> [w234 _]
              frame True {
                n83 = invoke class="VI" method="FP.Open"(reference=w235, error in=w236, "State"=w234) -> (error out=w237:errorcluster)  [unwired: 2 in, 4 out]
              }
              frame False {
              }
            }
          }
          frame "Maximize", "Maximized" {
            w239 = T12."Maximized" ("State")
            n84 = property class="VI"(reference=w245, error in=w244) -> (reference out=w242:refnum<vi>, error out=w243:errorcluster, "FP.State"=w241:T12)
            n85 = Not Equal?(x=w241, y=w239) -> (x != y?=w240:bool)
            n86 = case shown="True" w240 {
              tunnel: [w250 w251] -> w246
              tunnel: w243 -> [w249 w251]
              tunnel: w242 -> [w248 _]
              tunnel: w239 -> [w247 _]
              frame True {
                n87 = invoke class="VI" method="FP.Open"(reference=w248, error in=w249, "State"=w247) -> (error out=w250:errorcluster)  [unwired: 2 in, 4 out]
              }
              frame False {
              }
            }
          }
        }
        n88 = call <vilib>:"Add State(s) to Queue__JKI_lib_State_Machine.vi"("State(s) in (\"\")"=w186) -> ("States Out"=w185:string)  [unwired: 14 in]
      }
      frame "---------- Macro ----------" {
        # "Do not put any code in this frame.\n(It is a separator no-op. You can make a copy of this frame to create a new Macro frame)"
        n89 = call <vilib>:"Add State(s) to Queue__JKI_lib_State_Machine.vi"("State(s) in (\"\")"=w256) -> ("States Out"=w255:string)  [unwired: 14 in]
      }
      frame "Macro: Initialize" {
        # "Initialization Macro\n(This is called once, when the VI starts)"
        n90 = call <vilib>:"Add State(s) to Queue__JKI_lib_State_Machine.vi"("State(s) in Front (\"\")"="Data: Initialize\nInitialize Core Data\nEvents: Register\nUI: Initialize\nUI: Front Panel State >> Close\nFile Options: Read", "State(s) in (\"\")"=w262) -> ("States Out"=w261:string)  [unwired: 13 in]
      }
      frame "Macro: Exit" {
        # "Exit Macro\n(This is called once, when the VI exits)"
        n91 = Unbundle By Name(w270) -> ("Core.Close Panel on Exit?"=w269:bool)
        n92 = Select(t="UI: Front Panel State >> Close", s=w269, f="") -> (s? t:f=w266:string)
        n93 = call <vilib>:"Add State(s) to Queue__JKI_lib_State_Machine.vi"("State(s) in (\"\")"=w266, "State(s) at Back (\"\")"="Data: Cleanup\nEvents: Unregister\nExit") -> ("States Out"=w264:string)  [unwired: 13 in]
        n94 = call <vilib>:"Add State(s) to Queue__JKI_lib_State_Machine.vi"("State(s) in Front (\"\")"=w264, "State(s) in (\"\")"=w273) -> ("States Out"=w272:string)  [unwired: 13 in]
      }
      frame "---------- File Options ----------" {
        # "Template Separator\n(You can make a copy of, or modify, this frame)"
        n95 = call <vilib>:"Add State(s) to Queue__JKI_lib_State_Machine.vi"("State(s) in (\"\")"=w278) -> ("States Out"=w277:string)  [unwired: 14 in]
      }
      frame "File Options: Read" {
        # "Your code here.\n(You can make a copy of, or modify, this frame)"
        n96 = disable-structure shown="Enabled" {
          disable-tunnel: w280 -> [w291 w292]
          disable-tunnel: [w290 w292] -> w279
          frame Disabled {
            n97 = First Call?() -> (First Call?: T/F=w289:bool)
            n98 = Select(t=u32 800 ("milliseconds to wait"), s=w289, f=u32 0) -> (s? t:f=w287:u32)
            n99 = call "Stall Data Flow.vim"("value in"=w291, "milliseconds to wait"=w287) -> ("value out"=w290:errorcluster)  [unwired: 1 out]
          }
          frame Enabled {
          }
        }
        n100 = call "Send RefreshSystemConfigurationUI.vi"("error in (no error)"=w279, "Message Enqueuer"=w281) -> ()  [unwired: 8 in, 2 out]
        n101 = call <vilib>:"Add State(s) to Queue__JKI_lib_State_Machine.vi"("State(s) in (\"\")"=w285) -> ("States Out"=w284:string)  [unwired: 14 in]
      }
      frame "File Options: Write" {
        # "Your code here.\n(You can make a copy of, or modify, this frame)"
        n102 = call "Send SaveSystemConfigurationUI.vi"("Message Enqueuer"=w293) -> ()  [unwired: 9 in, 2 out]
        n103 = call <vilib>:"Add State(s) to Queue__JKI_lib_State_Machine.vi"("State(s) in (\"\")"=w298) -> ("States Out"=w297:string)  [unwired: 14 in]
      }
    }
  }
  n104 = call-parent "Actor Core.vi"("error in"="error in", "Actor in"=w12) -> ("error out"=→"error out":errorcluster, "Actor out"=→"HardwareSetup_modle001:HardwareSetup_modle001":refnum<class "Actor.lvclass">)  [unwired: 8 in]
